vi "CreateSavingCommand.vi"(8 "error in (no error)":errorcluster, 11 "StellarNet Black-Comet Spec in":refnum<class "StellarNet Black-Comet Spec.lvclass">) -> (0 "error out":errorcluster, 2 "NewCommandOut":string, 3 "StellarNet Black-Comet Spec out":refnum<class "StellarNet Black-Comet Spec.lvclass">)   [LabVIEW 2013, in "StellarNet Black-Comet Spec.lvclass"]
uses:
  StellarNet Black-Comet Spec.lvclass
  StellarNet Black-Comet Spec.lvclass/StellarNet Black-Comet Spec.ctl
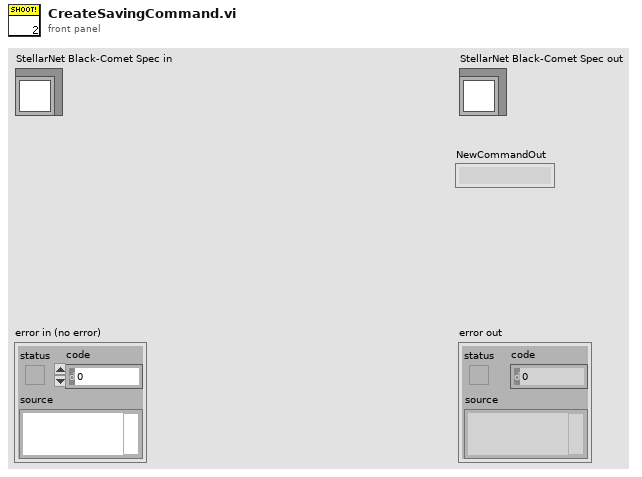
[diagram p1: front panel]
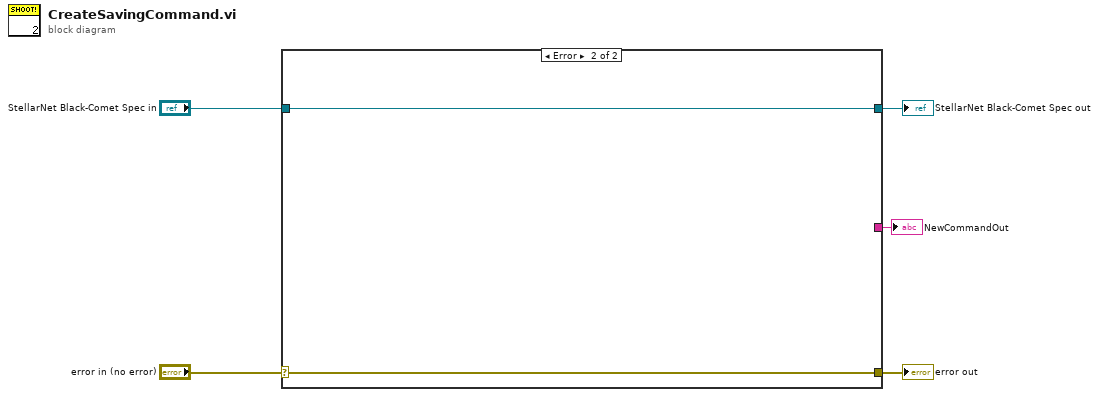
[diagram p0: block diagram]
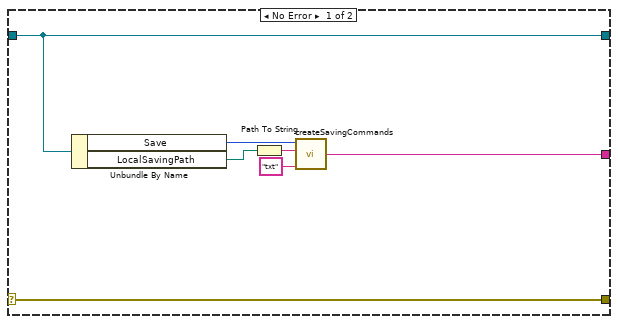
[diagram p2: hidden frame]
diagram:
  n1 = case shown="Error" "error in (no error)" {
    selector: "error in (no error)" -> [w12 w14]
    tunnel: [w12 w14] -> w4
    tunnel: [w7 w13] -> w2
    tunnel: "StellarNet Black-Comet Spec in" -> [w7 w13]
    tunnel: [w6 _] -> w1
    frame No Error {
      n2 = Unbundle By Name(w7) -> ("Save"=w9:enum16{"off", "on"}, "LocalSavingPath"=w8:path)
      n3 = Path To String(path=w8) -> (string=w10:string)
      n4 = call "createSavingCommands.vi"("extension"="txt" ("Fileextension"), "Saving Path (local)"=w10, "Save"=w9) -> ("String"=w6:string)  [unwired: 1 in]
    }
    frame Error {
    }
  }
  "error out" <- w4
  "StellarNet Black-Comet Spec out" <- w2
  "NewCommandOut" <- w1
